vi "Pasco Auton Drive Shoot.vi"(0 "Desired Heading":dbl, 1 "Actual Heading":dbl, 2 "time/distance":dbl, 3 "Power":dbl, 4 "Array":i32, 5 "Encoder total":dbl, 7 "Encoder Return":dbl) -> (14 "Left Drive":dbl, 15 "Right Drive":dbl, 16 "Array Out":i32, 17 "Encoder total":dbl)   [LabVIEW 2011]
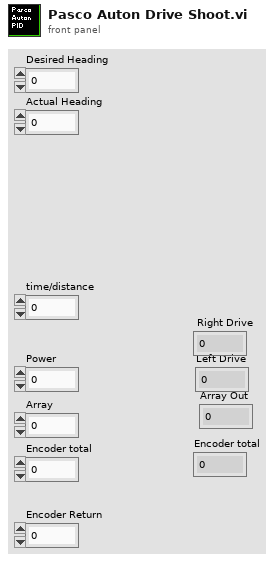
[diagram p1: front panel]
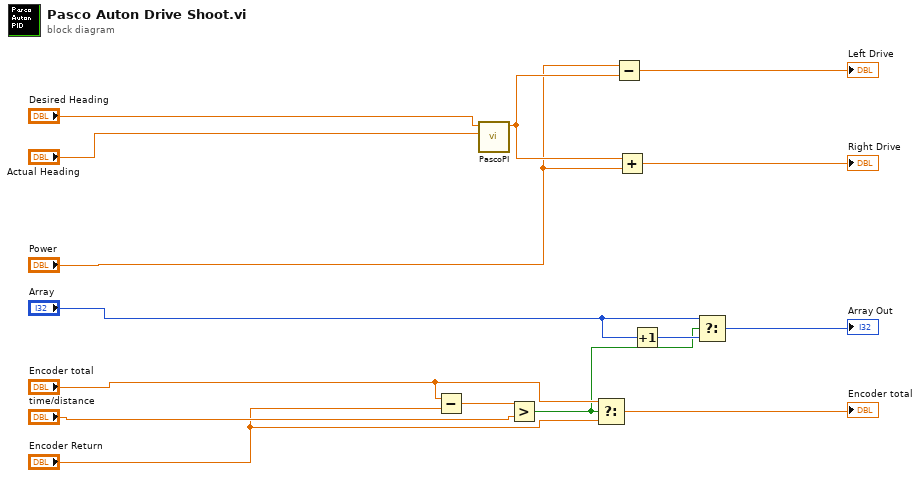
[diagram p0: block diagram]
diagram:
  n1 = Subtract(x="Encoder total", y="Encoder Return") -> (x-y=w15:dbl)
  n2 = call "PascoPI.vi"("Feedback"="Actual Heading", "Setpoint"="Desired Heading") -> ("Motor Output"=w14:dbl)  [unwired: 9 in]
  n3 = Greater?(x=w15, y="time/distance") -> (0:w6:bool)
  n4 = Select(t="Encoder total", s=w6, f="Encoder Return") -> (s? t:f=→"Encoder total":dbl)
  n5 = Subtract(x="Power", y=w14) -> (x-y=→"Left Drive":dbl)
  n6 = Add(x=w14, y="Power") -> (x+y=→"Right Drive":dbl)
  n7 = Increment(x="Array") -> (x+1=w7:i32)
  n8 = Select(t="Array", s=w6, f=w7) -> (s? t:f=→"Array Out":i32)
